vi "VideoOptStrToCode.vi"(7 "VideoOption":enum16{"FrameRate", "ImageType", "Resolution"}(ring), 8 "error in (no error)":errorcluster, 10 "DescriptionString":string, 11 "CameraTestingProxyAPI in":refnum<class "CameraTestingProxyAPI.lvclass">) -> (0 "error out":errorcluster, 2 "Code":u8, 3 "CameraTestingProxyAPI out":refnum<class "CameraTestingProxyAPI.lvclass">)   [LabVIEW 2020, in "CameraTestingProxy.lvlib" / "CameraTestingProxyAPI.lvclass"]
uses:
  CameraTestingProxyAPI.lvclass
  CameraTestingProxyAPI.lvclass/CameraTestingProxyAPI.ctl
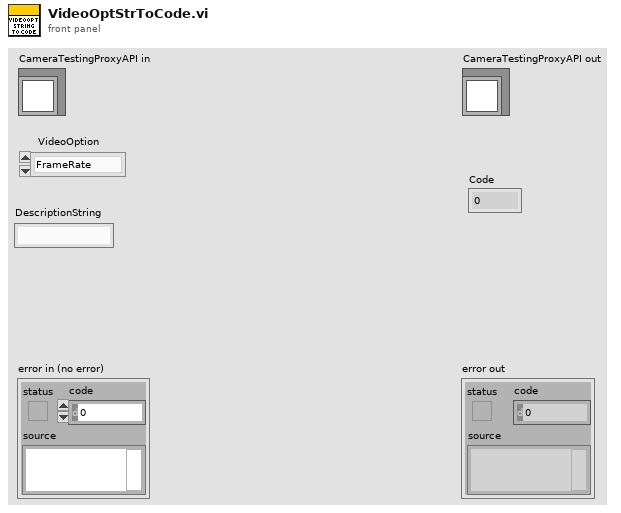
[diagram p1: front panel]
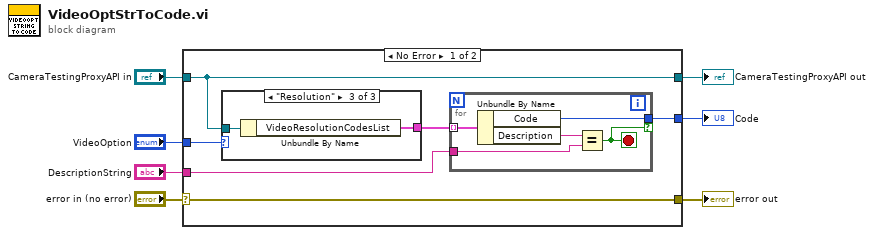
[diagram p0: block diagram]
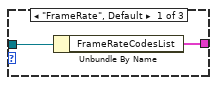
[diagram p2: hidden frame]
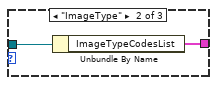
[diagram p3: hidden frame]
diagram:
  n1 = case shown="No Error" "error in (no error)" {
    selector: "error in (no error)" -> [w13 w26]
    tunnel: [w13 w26] -> w6
    tunnel: [w11 w25] -> w4
    tunnel: "CameraTestingProxyAPI in" -> [w11 w25]
    tunnel: "VideoOption" -> [w12 _]
    tunnel: "DescriptionString" -> [w9 _]
    tunnel: [w8 _] -> w1
    frame No Error {
      n2 = case shown="\"Resolution\"" w12 {
        tunnel: w11 -> [w20 w22 w24]
        tunnel: [w19 w21 w23] -> w10
        frame "FrameRate", Default {
          n3 = Unbundle By Name(w20) -> ("FrameRateCodesList"=w19:cluster{"Description":string, "Code":u8}[])
        }
        frame "ImageType" {
          n4 = Unbundle By Name(w22) -> ("ImageTypeCodesList"=w21:cluster{"Description":string, "Code":u8}[])
        }
        frame "Resolution" {
          n5 = Unbundle By Name(w24) -> ("VideoResolutionCodesList"=w23:cluster{"Description":string, "Code":u8}[])
        }
      }
      n6 = for {
        tunnel: w10 -> [w18] mode=indexing
        tunnel: w9 -> [w16]
        tunnel: [w15] -> w8 if=w14
        stop <- w14 stop-if-true
        n7 = Unbundle By Name(w18) -> ("Code"=w15:u8, "Description"=w17:string)
        n8 = Equal?(x=w17, y=w16) -> (x = y?=w14:bool)
      }
    }
    frame Error {
    }
  }
  "error out" <- w6
  "CameraTestingProxyAPI out" <- w4
  "Code" <- w1
